vi "gomokunarabe.vi"() -> ()   [LabVIEW 2022 SP3]
uses:
  moku.ctl
  <vilib>/Utility/miscctls.llb/LVPositionTypeDef.ctl
  <vilib>/Utility/miscctls.llb/LVBoundsTypeDef.ctl
  <vilib>/Utility/miscctls.llb/LVPoint32TypeDef.ctl
  <vilib>/Utility/miscctls.llb/LVPointTypeDef.ctl
  c_turn.ctl
panel:
  in  "game_Button":bool
  in  "Rule_Button":bool
  out "RULE/HOW TO USE":string="ETo Win\n    EAlign 5 same color pieces(stone). To align means vertical, horizontal, and diagonal.\n\nECondition \n    EBlack is first.\n    EEvery stones has quantum properties.\n    EYou don't know black or white until \"Observe\".\n    ELook right stones. Each stones number means probability to become black stone. Inversly, 10 stone is 90% to become white stone.\n    EYou can't choose 90 stone if your last turn choose 90 stone. 10 stone is also identical behavior.\n    EEach players can declare \"Observe\" 5 times.\n    EWhen a player declare \"Observe\" and both player could align, declaring player can win.\n\nEHow to use\n    EYou can click and select each right stone before you put a stone.\n    EAfter select, you can put stone on an arbitality cross point.\n"
  in  "CHKButton":bool
  in  "OvserveButton":bool
  out "index":i32[](array[numeric])
  out "Coords":T1
  out "Bounds":T2
  out "Position":T3
  in  "Send":bool
  in  "90b":bool
  in  "10b":bool
  in  "30b":bool
  in  "70b":bool
  out "Boolean":bool
  out "field":T4[][](array[typedef])
  out "pick":i32
  out "result":enum32{"black", "white", "none"}[][](array[radio])
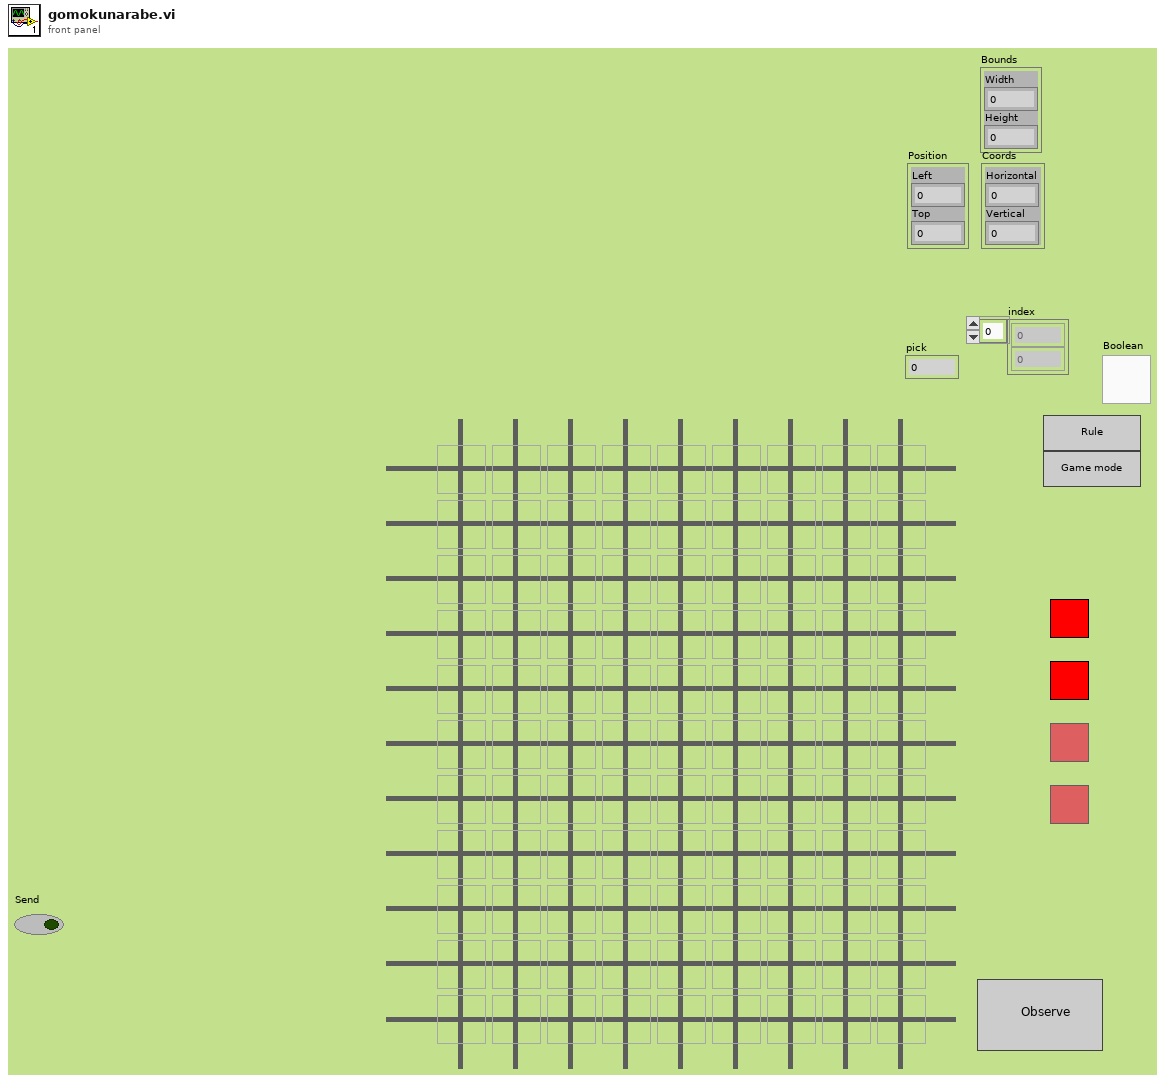
[diagram p1: front panel]
types:
  T1 = typedef "LVPoint32TypeDef.ctl" = cluster{"Horizontal":i32, "Vertical":i32}
  T2 = typedef "LVBoundsTypeDef.ctl" = cluster{"Width":u32, "Height":u32}
  T3 = typedef "LVPositionTypeDef.ctl" = cluster{"Left":i32, "Top":i32}
  T4 = typedef "moku.ctl" = enum32{"90b", "70b", "30b", "10b", "none"}
  T5 = typedef "c_turn.ctl" = enum16{"black", "white", "none"}
  T6 = typedef "LVPointTypeDef.ctl" = cluster{"Horizontal":i16, "Vertical":i16}
  T7 = enum8{"Enabled", "Disabled", "Disabled and Grayed Out"}
  T8 = enum32{"invalid app kind", "Development System", "Run Time System", "Student Edition", "Embedded LabVIEW", "Evaluation", "Custom"}
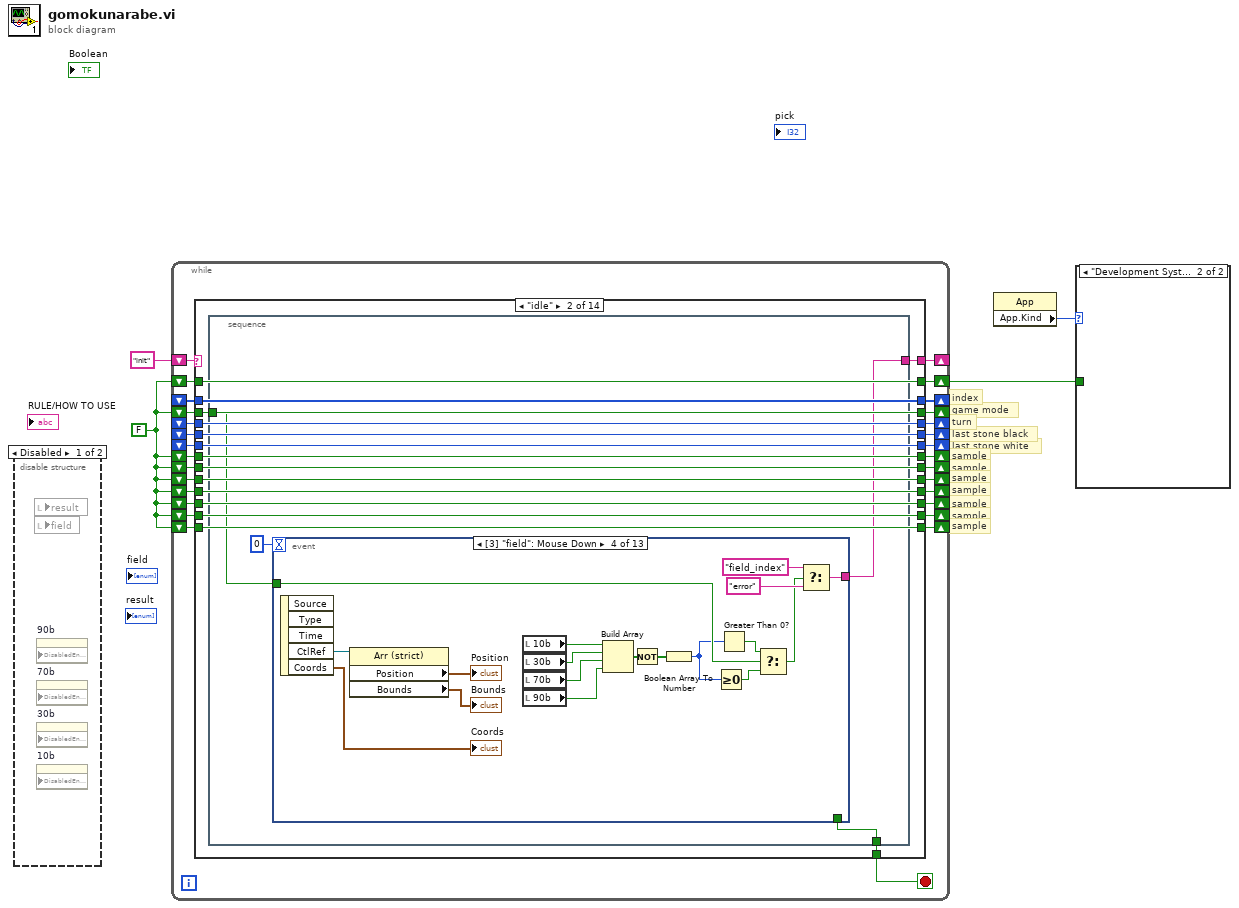
[diagram p0: block diagram]
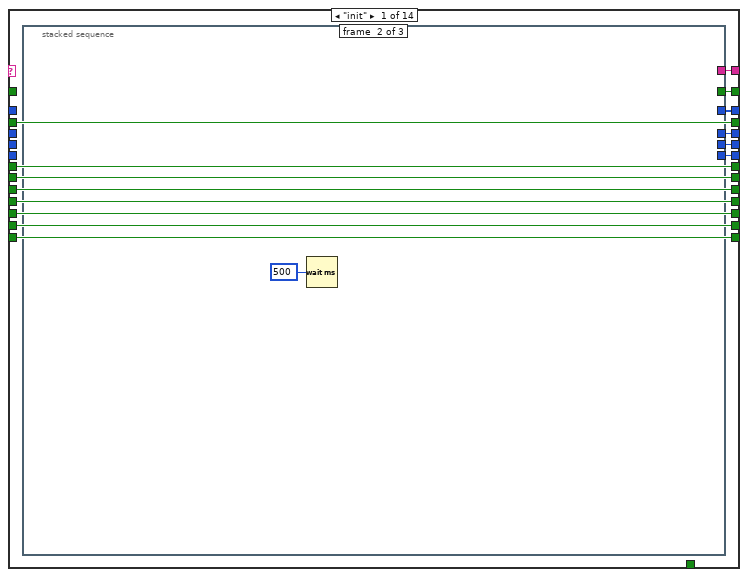
[diagram p3: hidden frame]
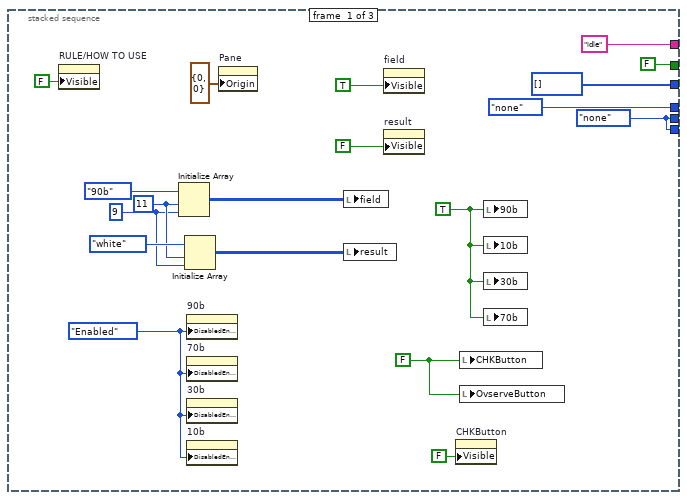
[diagram p4: hidden frame]
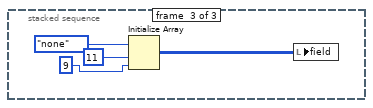
[diagram p5: hidden frame]
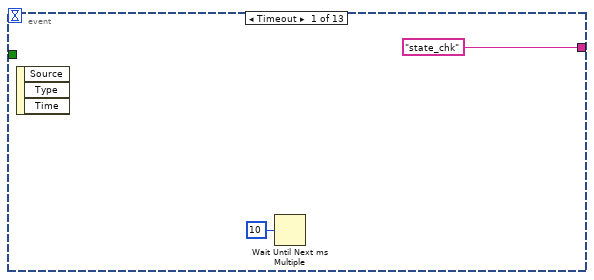
[diagram p6: hidden frame]
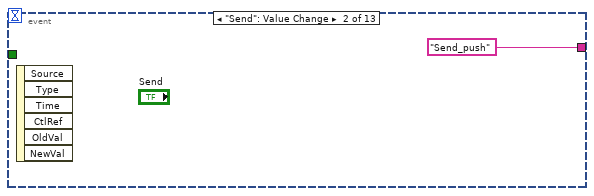
[diagram p7: hidden frame]
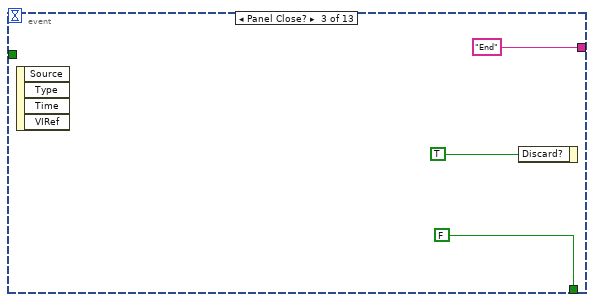
[diagram p8: hidden frame]
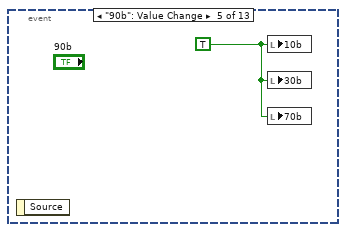
[diagram p9: hidden frame]
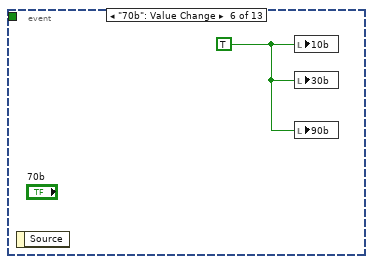
[diagram p10: hidden frame]
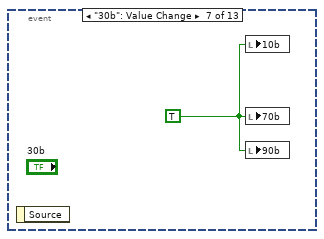
[diagram p11: hidden frame]
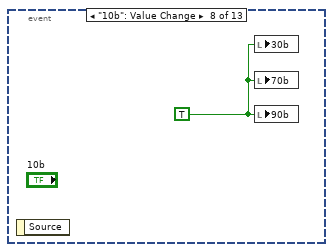
[diagram p12: hidden frame]
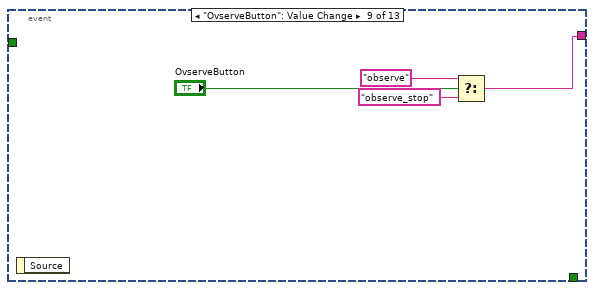
[diagram p13: hidden frame]
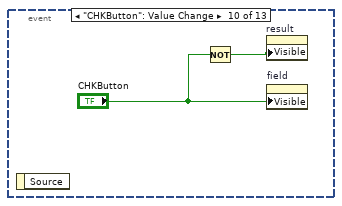
[diagram p14: hidden frame]
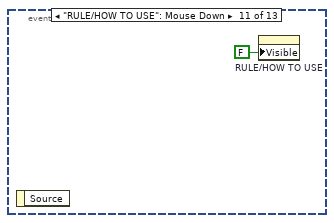
[diagram p15: hidden frame]
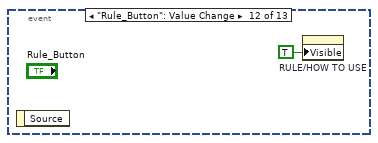
[diagram p16: hidden frame]
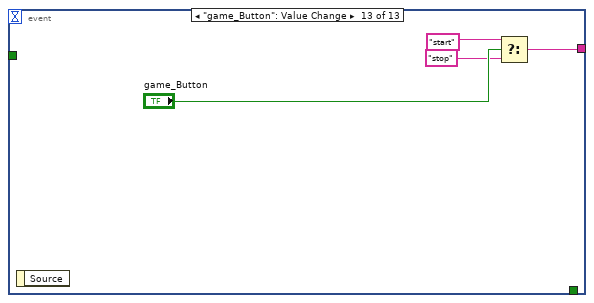
[diagram p17: hidden frame]
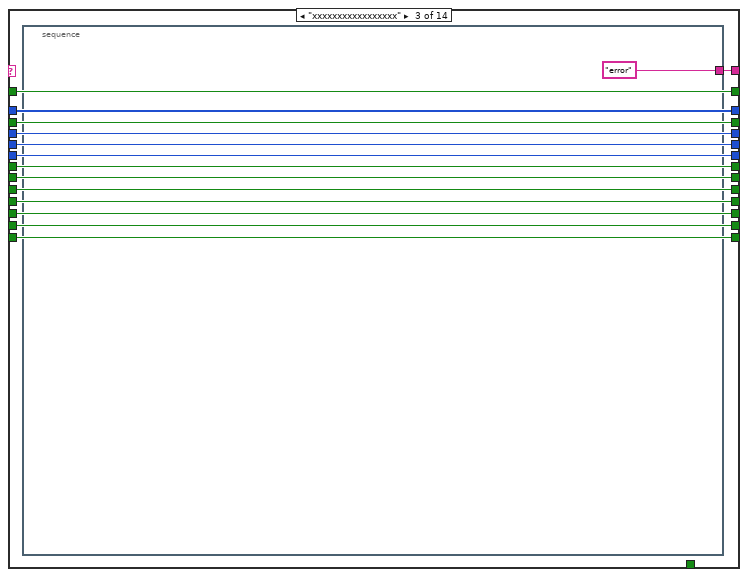
[diagram p18: hidden frame]
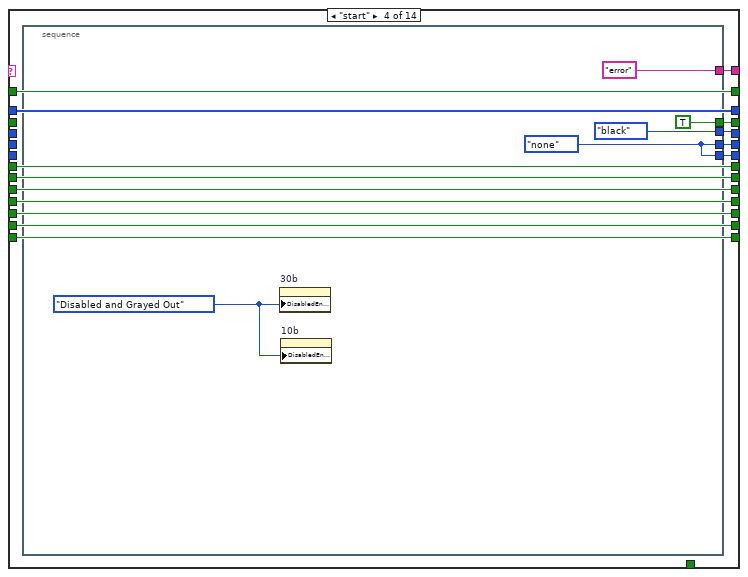
[diagram p19: hidden frame]
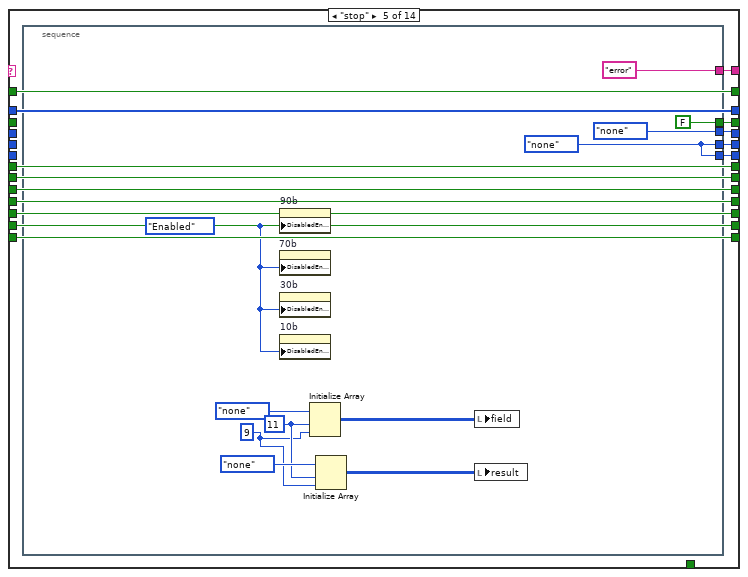
[diagram p20: hidden frame]
diagram:
  w1 = FALSE
  # "index"
  # "game mode"
  # "turn"
  # "last stone black"
  # "last stone white"
  # "sample"
  # "sample"
  # "sample"
  # "sample"
  # "sample"
  # "sample"
  # "sample"
  n1 = disable-structure shown="Disabled" {
    frame Disabled {
      n2 = local read "result"() -> ()  [unwired: 1 in]
      n3 = local read "field"() -> ()  [unwired: 1 in]
      n4 = property on="90b" class="Bool (strict)" props=["DisabledEnum"]() -> ()  [unwired: 3 in, 2 out]
      n5 = property on="70b" class="Bool (strict)" props=["DisabledEnum"]() -> ()  [unwired: 3 in, 2 out]
      n6 = property on="30b" class="Bool (strict)" props=["DisabledEnum"]() -> ()  [unwired: 3 in, 2 out]
      n7 = property on="10b" class="Bool (strict)" props=["DisabledEnum"]() -> ()  [unwired: 3 in, 2 out]
    }
    frame Enabled {
    }
  }
  n8 = while {
    shift-right: [w32] -> _
    shift-left: "init" -> [w33]
    shift-right: [w30] -> w3
    shift-left: w1 -> [w29]
    shift-right: [w27] -> _
    shift-left: _ -> [w28]
    shift-right: [w26] -> _
    shift-left: w1 -> [w25]
    shift-right: [w23] -> _
    shift-left: _ -> [w24]
    shift-right: [w22] -> _
    shift-left: _ -> [w21]
    shift-right: [w19] -> _
    shift-left: _ -> [w20]
    shift-right: [w18] -> _
    shift-left: w1 -> [w17]
    shift-right: [w15] -> _
    shift-left: w1 -> [w16]
    shift-right: [w14] -> _
    shift-left: w1 -> [w13]
    shift-right: [w11] -> _
    shift-left: w1 -> [w12]
    shift-right: [w10] -> _
    shift-left: w1 -> [w9]
    shift-right: [w7] -> _
    shift-left: w1 -> [w8]
    shift-right: [w6] -> _
    shift-left: w1 -> [w5]
    stop <- w31 stop-if-true
    n9 = case shown="\"idle\"" w33 {
      tunnel: [w47 w86 w144 w159 w178 w203 w218 w275 w321 w364 w384 w403 w418 w434] -> w32
      tunnel: [_ w85 _ _ _ _ _ _ _ _ _ _ _ w432] -> w31
      tunnel: [w38 w84 w143 w158 w177 w202 w217 w274 w320 w363 w383 w402 w417 w433] -> w30
      tunnel: w29 -> [_ w84 w143 w158 w177 w202 w217 w274 w320 w363 w383 w402 w417 w433]
      tunnel: w28 -> [_ w73 w142 w157 w176 w201 _ w266 w319 w362 w382 w401 w416 w431]
      tunnel: [w37 w73 w142 w157 w176 w201 w205 w266 w319 w362 w382 w401 w416 w431] -> w27
      tunnel: w25 -> [w46 w72 w141 _ _ w200 w216 w265 w318 w361 w381 w400 w415 w430]
      tunnel: [w46 w72 w141 w149 w168 w200 w216 w265 w318 w361 w381 w400 w415 w430] -> w26
      tunnel: w24 -> [_ w83 w140 _ _ w199 w215 w264 w310 w360 w380 w399 w414 w429]
      tunnel: [w36 w83 w140 w148 w167 w199 w215 w264 w308 w360 w380 w399 w414 w429] -> w23
      tunnel: w21 -> [_ w82 w139 _ _ w198 w214 w263 w309 w359 w379 w398 w413 w428]
      tunnel: [w35 w82 w139 w147 w166 w198 w214 w261 w309 w359 w379 w398 w413 w428] -> w22
      tunnel: w20 -> [_ w81 w138 _ _ w197 w213 w262 w307 w358 w378 w397 w412 w427]
      tunnel: [w34 w81 w138 w146 w165 w197 w213 w260 w307 w358 w378 w397 w412 w427] -> w19
      tunnel: w17 -> [w45 w80 w137 w156 w175 w196 w212 w273 w317 w357 w377 w396 w411 w426]
      tunnel: [w45 w80 w137 w156 w175 w196 w212 w273 w317 w357 w377 w396 w411 w426] -> w18
      tunnel: w16 -> [w44 w79 w136 w155 w174 w195 w211 w272 w316 w356 w376 w395 w410 w425]
      tunnel: [w44 w79 w136 w155 w174 w195 w211 w272 w316 w356 w376 w395 w410 w425] -> w15
      tunnel: w13 -> [w43 w78 w135 w154 w173 w194 w210 w271 w315 w355 w375 w394 w409 w424]
      tunnel: [w43 w78 w135 w154 w173 w194 w210 w271 w315 w355 w375 w394 w409 w424] -> w14
      tunnel: w12 -> [w42 w77 w134 w153 w172 w193 w209 w270 w314 w354 w374 w393 w408 w423]
      tunnel: [w42 w77 w134 w153 w172 w193 w209 w270 w314 w354 w374 w393 w408 w423] -> w11
      tunnel: w9 -> [w41 w76 w133 w152 w171 w192 w208 w269 w313 w353 w373 w392 w407 w422]
      tunnel: [w41 w76 w133 w152 w171 w192 w208 w269 w313 w353 w373 w392 w407 w422] -> w10
      tunnel: w8 -> [w40 w75 w132 w151 w170 w191 w207 w268 w312 w352 w372 w391 w406 w421]
      tunnel: [w40 w75 w132 w151 w170 w191 w207 w268 w312 w352 w372 w391 w406 w421] -> w7
      tunnel: w5 -> [w39 w74 w131 w150 w169 w190 w206 w267 w311 w351 w371 w390 w405 w420]
      tunnel: [w39 w74 w131 w150 w169 w190 w206 w267 w311 w351 w371 w390 w405 w420] -> w6
      frame "init" {
        n10 = stacked-sequence {
          tunnel: ["idle" _ _] -> w47
          tunnel: [FALSE _ _] -> w38
          tunnel: [i32[] [] _ _] -> w37
          tunnel: [c_turn."none" ("turn") _ _] -> w36
          tunnel: [w49 _ _] -> w35
          tunnel: [w49 _ _] -> w34
          frame #0 {
            w48 = T7."Enabled" ("Disabled")
            w49 = moku."none" ("new element/subarray")
            w52 = FALSE ("CHKButton")
            w54 = TRUE ("90b")
            w62 = 9 ("dimension size")
            w63 = 11 ("dimension size")
            n11 = property on="RULE/HOW TO USE" class="Str"("Visible"=FALSE) -> ()  [unwired: 2 in, 2 out]
            n12 = Initialize Array(moku."90b" ("moku"), w63, w62) -> (w58:T4[][])
            n13 = Initialize Array(enum32{"black", "white", "none"}."white" ("black/white"), w63, w62) -> (w57:enum32{"black", "white", "none"}[][])
            n14 = property on="90b" class="Bool (strict)"("DisabledEnum"=w48) -> ()  [unwired: 2 in, 2 out]
            n15 = property on="70b" class="Bool (strict)"("DisabledEnum"=w48) -> ()  [unwired: 2 in, 2 out]
            n16 = property on="30b" class="Bool (strict)"("DisabledEnum"=w48) -> ()  [unwired: 2 in, 2 out]
            n17 = property on="10b" class="Bool (strict)"("DisabledEnum"=w48) -> ()  [unwired: 2 in, 2 out]
            n18 = property on="Pane" class="Pane"("Origin"=T6 {"Horizontal"=0, "Vertical"=0}) -> ()  [unwired: 2 in, 2 out]
            n19 = local write "field"(w58) -> ()
            n20 = local write "result"(w57) -> ()
            n21 = property on="field" class="Arr (strict)"("Visible"=TRUE) -> ()  [unwired: 2 in, 2 out]
            n22 = property on="result" class="Arr (strict)"("Visible"=FALSE) -> ()  [unwired: 2 in, 2 out]
            n23 = property on="CHKButton" class="Bool (strict)"("Visible"=FALSE) -> ()  [unwired: 2 in, 2 out]
            n24 = local write "CHKButton"(w52) -> ()
            n25 = local write "OvserveButton"(w52) -> ()
            n26 = local write "90b"(w54) -> ()
            n27 = local write "10b"(w54) -> ()
            n28 = local write "30b"(w54) -> ()
            n29 = local write "70b"(w54) -> ()
          }
          frame #1 {
            n30 = Wait (ms)(milliseconds to wait=u32 500) -> ()  [unwired: 1 out]
          }
          frame #2 {
            n31 = Initialize Array(moku."none" ("moku"), 11 ("dimension size"), 9 ("dimension size")) -> (w71:T4[][])
            n32 = local write "field"(w71) -> ()
          }
        }
      }
      frame "idle" {
        n33 = stacked-sequence {
          tunnel: [w89] -> w86
          tunnel: [w88] -> w85
          tunnel: w72 -> [w87]
          frame #0 {
            n34 = event shown="[3] \"field\": Mouse Down" {
              selector: _ -> [_ _ _ _ _ _ _ _ _ _ _ _ _]
              dyn-events: _ -> [_ _ _ _ _ _ _ _ _ _ _ _ _]
              timeout: 0 -> [_ _ _ _ _ _ _ _ _ _ _ _ _]
              tunnel: ["state_chk" "Send_push" "End" w102 _ _ _ _ w119 _ _ _ w127] -> w89
              tunnel: [_ _ FALSE ("Discard?") _ _ _ _ _ _ _ _ _ _] -> w88
              tunnel: w87 -> [_ _ _ w101 _ _ _ _ _ _ _ _ _]
              event Timeout {
                n35 = event-data() -> ()  [unwired: 1 in, 3 out]
                n36 = Wait Until Next ms Multiple(millisecond multiple=u32 10) -> ()  [unwired: 1 out]
              }
              event "Send": Value Change {
                n37 = event-data() -> ()  [unwired: 1 in, 6 out]
              }
              event Panel Close? {
                n38 = event-data() -> ()  [unwired: 1 in, 4 out]
                n39 = event-data("Discard?"=TRUE) -> ()  [unwired: 1 in, 1 out]
              }
              event "field": Mouse Down {
                n40 = event-data() -> ("CtlRef"=w114:refnum<vi>, "Coords"=→"Coords":T1)  [unwired: 1 in, 3 out]
                n41 = property on="Property Node" class="Arr (strict)"(reference=w114) -> ("Position"=→"Position":T3, "Bounds"=→"Bounds":T2)  [unwired: 1 in, 2 out]
                n42 = local read "10b"() -> (w110:bool)
                n43 = local read "30b"() -> (w109:bool)
                n44 = local read "70b"() -> (w108:bool)
                n45 = local read "90b"() -> (w107:bool)
                n46 = Build Array(w110, w109, w108, w107) -> (w106:bool[])
                n47 = Not(x=w106) -> (.not. x?=w105:bool[])
                n48 = Boolean Array To Number(Boolean array=w105) -> (number=w98:u32)
                n49 = Greater Or Equal To 0?(x=w98) -> (x >= 0?=w97:bool)
                n50 = Greater Than 0?(x=w98) -> (x > 0?=w99:bool)
                n51 = Select(t=w99, s=w101, f=w97) -> (s? t:f=w100:bool)
                n52 = Select(t="field_index", s=w100, f="error") -> (s? t:f=w102:string)
              }
              event "90b": Value Change {
                w115 = TRUE ("10b")
                n53 = event-data() -> ()  [unwired: 1 in, 1 out]
                n54 = local write "10b"(w115) -> ()
                n55 = local write "30b"(w115) -> ()
                n56 = local write "70b"(w115) -> ()
              }
              event "70b": Value Change {
                w116 = TRUE ("10b")
                n57 = event-data() -> ()  [unwired: 1 in, 1 out]
                n58 = local write "10b"(w116) -> ()
                n59 = local write "30b"(w116) -> ()
                n60 = local write "90b"(w116) -> ()
              }
              event "30b": Value Change {
                w117 = TRUE ("70b")
                n61 = event-data() -> ()  [unwired: 1 in, 1 out]
                n62 = local write "10b"(w117) -> ()
                n63 = local write "70b"(w117) -> ()
                n64 = local write "90b"(w117) -> ()
              }
              event "10b": Value Change {
                w118 = TRUE ("90b")
                n65 = event-data() -> ()  [unwired: 1 in, 1 out]
                n66 = local write "30b"(w118) -> ()
                n67 = local write "70b"(w118) -> ()
                n68 = local write "90b"(w118) -> ()
              }
              event "OvserveButton": Value Change {
                n69 = event-data() -> ()  [unwired: 1 in, 1 out]
                n70 = Select(t="observe", s="OvserveButton", f="observe_stop") -> (s? t:f=w119:string)
              }
              event "CHKButton": Value Change {
                n71 = event-data() -> ()  [unwired: 1 in, 1 out]
                n72 = Not(x="CHKButton") -> (.not. x?=w123:bool)
                n73 = property on="result" class="Arr (strict)"("Visible"=w123) -> ()  [unwired: 2 in, 2 out]
                n74 = property on="field" class="Arr (strict)"("Visible"="CHKButton") -> ()  [unwired: 2 in, 2 out]
              }
              event "RULE/HOW TO USE": Mouse Down {
                n75 = event-data() -> ()  [unwired: 1 in, 1 out]
                n76 = property on="RULE/HOW TO USE" class="Str"("Visible"=FALSE) -> ()  [unwired: 2 in, 2 out]
              }
              event "Rule_Button": Value Change {
                n77 = event-data() -> ()  [unwired: 1 in, 1 out]
                n78 = property on="RULE/HOW TO USE" class="Str"("Visible"=TRUE) -> ()  [unwired: 2 in, 2 out]
              }
              event "game_Button": Value Change {
                n79 = event-data() -> ()  [unwired: 1 in, 1 out]
                n80 = Select(t="start" ("f"), s="game_Button", f="stop") -> (s? t:f=w127:string)
              }
            }
          }
        }
      }
      frame "xxxxxxxxxxxxxxxxx" {
        n81 = stacked-sequence {
          tunnel: ["error"] -> w144
          frame #0 {
          }
        }
      }
      frame "start" {
        n82 = stacked-sequence {
          tunnel: ["error"] -> w159
          tunnel: [TRUE] -> w149
          tunnel: [c_turn."black" ("turn")] -> w148
          tunnel: [w160] -> w147
          tunnel: [w160] -> w146
          frame #0 {
            w160 = moku."none" ("new element/subarray")
            w161 = T7."Disabled and Grayed Out" ("Disabled")
            n83 = property on="30b" class="Bool (strict)"("DisabledEnum"=w161) -> ()  [unwired: 2 in, 2 out]
            n84 = property on="10b" class="Bool (strict)"("DisabledEnum"=w161) -> ()  [unwired: 2 in, 2 out]
          }
        }
      }
      frame "stop" {
        n85 = stacked-sequence {
          tunnel: ["error"] -> w178
          tunnel: [FALSE] -> w168
          tunnel: [c_turn."none" ("turn")] -> w167
          tunnel: [w186] -> w166
          tunnel: [w186] -> w165
          frame #0 {
            w180 = 9 ("dimension size")
            w181 = 11 ("dimension size")
            w186 = moku."none" ("new element/subarray")
            w185 = T7."Enabled" ("Disabled")
            n86 = property on="90b" class="Bool (strict)"("DisabledEnum"=w185) -> ()  [unwired: 2 in, 2 out]
            n87 = property on="70b" class="Bool (strict)"("DisabledEnum"=w185) -> ()  [unwired: 2 in, 2 out]
            n88 = property on="30b" class="Bool (strict)"("DisabledEnum"=w185) -> ()  [unwired: 2 in, 2 out]
            n89 = property on="10b" class="Bool (strict)"("DisabledEnum"=w185) -> ()  [unwired: 2 in, 2 out]
            n90 = Initialize Array(moku."none" ("moku"), w181, w180) -> (w184:T4[][])
            n91 = Initialize Array(enum32{"black", "white", "none"}."none" ("black/white"), w181, w180) -> (w183:enum32{"black", "white", "none"}[][])
            n92 = local write "field"(w184) -> ()
            n93 = local write "result"(w183) -> ()
          }
        }
      }
      frame "state_chk" {
        n94 = stacked-sequence {
          tunnel: ["error"] -> w203
          frame #0 {
          }
        }
      }
      frame "field_index" {
        n95 = stacked-sequence {
          tunnel: ["field_change"] -> w218
          tunnel: [w219] -> w205
          frame #0 {
            n96 = local read "Position"() -> (w224:T3)
            n97 = local read "Bounds"() -> (w223:T2)
            n98 = local read "Coords"() -> (w222:T1)
            n99 = property on="field" class="Arr (strict)"() -> ("Number of Rows"=w221:u32, "Number of Columns"=w220:u32)  [unwired: 2 in, 2 out]
            n100 = Unbundle By Name(w223) -> ("Width"=w231:u32, "Height"=w232:u32)
            n101 = Unbundle By Name(w222) -> ("Horizontal"=w233:i32, "Vertical"=w234:i32)
            n102 = Unbundle By Name(w224) -> ("Left"=w229:i32, "Top"=w230:i32)
            n103 = Build Array(w230, w229) -> (w228:i32[])
            n104 = Build Array(w232, w231) -> (w226:u32[])
            n105 = Build Array(w234, w233) -> (w227:i32[])
            n106 = Build Array(w221, w220) -> (w235:u32[])
            n107 = Divide(x=w226, y=w235) -> (x/y=w236:dbl[])
            n108 = for {
              N: 2 -> [_]
              tunnel: w227 -> [w242] mode=indexing
              tunnel: w236 -> [w241] mode=indexing
              tunnel: w228 -> [w240] mode=indexing
              tunnel: [w239] -> w219 mode=indexing
              tunnel: w235 -> [w238] mode=indexing
              n109 = while {
                tunnel: w242 -> [w243]
                tunnel: w241 -> [w249]
                tunnel: w240 -> [w245]
                tunnel: [w254] -> w239
                tunnel: w238 -> [w244]
                i -> [w248]
                stop <- w252 stop-if-true
                n110 = Increment(x=w248) -> (x+1=w259:i32)
                n111 = Multiply(x=w249, y=w248) -> (x*y=w246:dbl)
                n112 = Multiply(x=w249, y=w259) -> (x*y=w257:dbl)
                n113 = Add(x=w245, y=w246) -> (x+y=w247:dbl)
                n114 = Add(x=w245, y=w257) -> (x+y=w258:dbl)
                n115 = Greater Or Equal?(x=w243, y=w247) -> (x >= y?=w256:bool)
                n116 = Less Or Equal?(x=w243, y=w258) -> (x <= y?=w255:bool)
                n117 = And(x=w256, y=w255) -> (x .and. y?=w251:bool)
                n118 = Greater?(x=w248, y=w244) -> (0:w250:bool)
                n119 = Or(x=w251, y=w250) -> (x .or. y?=w252:bool)
                n120 = Select(t=w248, s=w251, f=-1) -> (s? t:f=w254:i32)
              }
            }
          }
        }
      }
      frame "field_change" {
        n121 = stacked-sequence {
          tunnel: [w282] -> w275
          tunnel: w266 -> [w286]
          tunnel: w265 -> [w284]
          tunnel: w264 -> [w281]
          tunnel: w263 -> [w280]
          tunnel: w262 -> [w279]
          tunnel: [w277] -> w261
          tunnel: [w276] -> w260
          frame #0 {
            n122 = local read "90b"() -> (w297:bool)
            n123 = local read "70b"() -> (w296:bool)
            n124 = local read "30b"() -> (w295:bool)
            n125 = local read "10b"() -> (w294:bool)
            n126 = Index Array(array=w286) -> (element #1=w291:i32, element #2=w290:i32)  [unwired: 2 in]
            n127 = Build Array(w297, w296, w295, w294) -> (w293:bool[])
            n128 = Not(x=w293) -> (.not. x?=w287:bool[])
            n129 = Boolean Array To Number(Boolean array=w287) -> (number=w289:u32)
            n130 = case shown="0, Default" w289 {
              tunnel: [moku."none" ("new element/subarray") moku."90b" ("new element/subarray") moku."70b" ("new element/subarray") moku."30b" ("new element/subarray") moku."10b" ("new element/subarray")] -> w278
              frame 0, Default {
              }
              frame 1 {
              }
              frame 2 {
              }
              frame 4 {
              }
              frame 8 {
              }
            }
            n131 = local read "field"() -> (w292:T4[][])
            n132 = case shown="\"black\", Default" w281 {
              tunnel: w280 -> [_ w300]
              tunnel: w279 -> [w298 _]
              tunnel: w278 -> [w299 w301]
              tunnel: [w299 w300] -> w277
              tunnel: [w298 w301] -> w276
              frame "black", Default {
              }
              frame "white" {
              }
            }
            n133 = Replace Array Subset(array=w292, new element=w278, index (row)=w291, index (col)=w290) -> (w288:T4[][])
            n134 = local write "field"(w288) -> ()
            n135 = Select(t="stone_chk", s=w284, f="error") -> (s? t:f=w282:string)
            "index" <- w286
          }
        }
      }
      frame "stone_chk" {
        n136 = stacked-sequence {
          tunnel: ["error"] -> w321
          tunnel: w310 -> [w330]
          tunnel: w309 -> [w323]
          tunnel: [w325] -> w308
          tunnel: w307 -> [w324]
          frame #0 {
            w322 = TRUE ("10b")
            n137 = case shown="\"black\", Default" w330 {
              tunnel: [T7."Disabled and Grayed Out" ("Disabled") w342] -> w329
              tunnel: [T7."Enabled" ("Disabled") w348] -> w328
              tunnel: [T7."Disabled and Grayed Out" ("Disabled") T7."Enabled" ("Disabled")] -> w327
              tunnel: w324 -> [w337 _]
              tunnel: [w333 w348] -> w326
              tunnel: [c_turn."white" ("turn") c_turn."black" ("turn")] -> w325
              tunnel: w323 -> [_ w343]
              frame "black", Default {
                n138 = Equal?(x=w337, y=moku."10b" ("new element/subarray")) -> (x = y?=w336:bool)
                n139 = Select(t=T7."Disabled and Grayed Out" ("Disabled"), s=w336, f=T7."Enabled") -> (s? t:f=w333:T7)
              }
              frame "white" {
                w348 = T7."Disabled and Grayed Out" ("Disabled")
                n140 = Equal?(x=w343, y=moku."90b" ("new element/subarray")) -> (x = y?=w346:bool)
                n141 = Select(t=T7."Disabled and Grayed Out" ("Disabled"), s=w346, f=T7."Enabled") -> (s? t:f=w342:T7)
              }
            }
            n142 = property on="90b" class="Bool (strict)"("DisabledEnum"=w329) -> ()  [unwired: 2 in, 2 out]
            n143 = property on="70b" class="Bool (strict)"("DisabledEnum"=w327) -> ()  [unwired: 2 in, 2 out]
            n144 = property on="30b" class="Bool (strict)"("DisabledEnum"=w328) -> ()  [unwired: 2 in, 2 out]
            n145 = property on="10b" class="Bool (strict)"("DisabledEnum"=w326) -> ()  [unwired: 2 in, 2 out]
            n146 = local write "10b"(w322) -> ()
            n147 = local write "30b"(w322) -> ()
            n148 = local write "70b"(w322) -> ()
            n149 = local write "90b"(w322) -> ()
          }
        }
      }
      frame "observe" {
        n150 = stacked-sequence {
          tunnel: [_ "error" _] -> w364
          frame #0 {
            w366 = FALSE ("Visible")
            n151 = property on="field" class="Arr (strict)"("Visible"=w366) -> ()  [unwired: 2 in, 2 out]
            n152 = property on="result" class="Arr (strict)"("Visible"=w366) -> ()  [unwired: 2 in, 2 out]
            n153 = property on="CHKButton" class="Bool (strict)"("Visible"=TRUE) -> ()  [unwired: 2 in, 2 out]
          }
          frame #1 {
            n154 = local read "field"() -> (w368:T4[][])
            n155 = call "prob.vi"("field"=w368) -> ("result"=w367:enum32{"black", "white", "none"}[][])  [unwired: 10 in]
            n156 = local write "result"(w367) -> ()
          }
          frame #2 {
            n157 = property on="result" class="Arr (strict)"("Visible"=TRUE) -> ()  [unwired: 2 in, 2 out]
          }
        }
      }
      frame "observe_stop" {
        n158 = stacked-sequence {
          tunnel: ["error"] -> w384
          frame #0 {
            n159 = local write "CHKButton"(FALSE ("CHKButton")) -> ()
            n160 = property on="CHKButton" class="Bool (strict)"("Visible"=FALSE) -> ()  [unwired: 2 in, 2 out]
            n161 = property on="field" class="Arr (strict)"("Visible"=TRUE) -> ()  [unwired: 2 in, 2 out]
            n162 = property on="result" class="Arr (strict)"("Visible"=FALSE) -> ()  [unwired: 2 in, 2 out]
          }
        }
      }
      frame "error", Default {
        n163 = stacked-sequence {
          tunnel: ["idle"] -> w403
          frame #0 {
          }
        }
      }
      frame "End" {
        n164 = stacked-sequence {
          tunnel: ["Fin"] -> w418
          tunnel: w417 -> [_]
          frame #0 {
          }
        }
      }
      frame "Fin" {
        n165 = stacked-sequence {
          tunnel: [_ "Fin"] -> w434
          tunnel: w433 -> [_ _]
          tunnel: [_ TRUE] -> w432
          frame #0 {
            n166 = Wait Until Next ms Multiple(millisecond multiple=u32 1000) -> ()  [unwired: 1 out]
          }
          frame #1 {
          }
        }
      }
    }
  }
  n167 = property class="App"() -> ("App.Kind"=w2:T8)  [unwired: 2 in, 2 out]
  n168 = case shown="\"Development System\"" w2 {
    tunnel: w3 -> [w438 _]
    frame Default {
      n169 = flat-sequence {
        tunnel: w438 -> [_]
        frame #0 {
          n170 = Quit LabVIEW(quit? (T)=TRUE) -> ()
        }
      }
    }
    frame "Development System" {
    }
  }
